vi "Destructor.vi"(8 "ErrorIn":errorcluster, 11 "OpenCVCamIn":refnum<class "OpenCVCam.lvclass">) -> (0 "ErrorOut":errorcluster, 3 "OpenCVCamOut":refnum<class "OpenCVCam.lvclass">)   [LabVIEW 2021, in "OpenCVCam.lvclass"]
doc: "Called at the destruction of the object. Use this to clear references or perform action to tidy up the object."
uses:
  OpenCVCam.lvclass
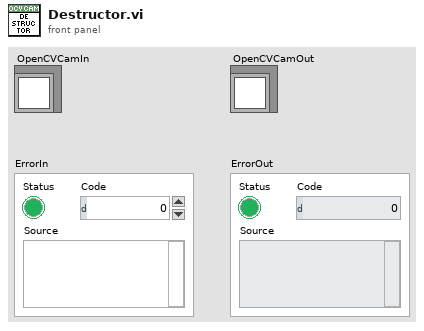
[diagram p1: front panel]
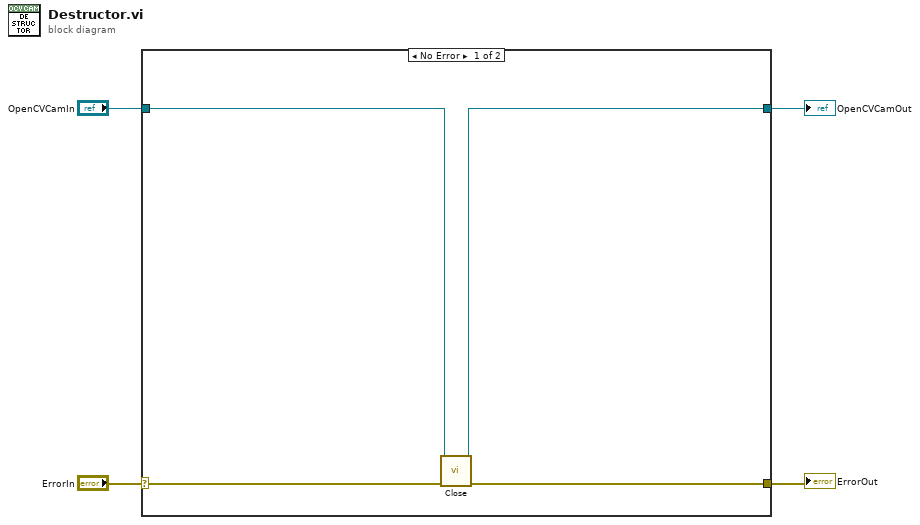
[diagram p0: block diagram]
diagram:
  n1 = case shown="No Error" "ErrorIn" {
    selector: "ErrorIn" -> [w8 w10]
    tunnel: [w7 w10] -> w3
    tunnel: [w5 w9] -> w1
    tunnel: "OpenCVCamIn" -> [w6 w9]
    frame No Error {
      n2 = call-dynamic "Close.vi"("ErrorIn"=w8, "OpenCVCamIn"=w6) -> ("ErrorOut"=w7:errorcluster, "OpenCVCamOut"=w5:refnum<class "OpenCVCam.lvclass">)  [unwired: 8 in]
    }
    frame Error {
    }
  }
  "ErrorOut" <- w3
  "OpenCVCamOut" <- w1
